vi "OE2012&OE2022_Query Multi Data.vi"(0 "VISA resource name":refnum<visa-resource-name>, 1 "OE2012&OE2022_\nQuery Multi Data":T2={"Query Type 1"=0, "Query Type 5"=32, "Query Type 4"=3, "Query Type 3"=2, "Query Type 2"=1, "Query Type 6"=36} {"Query Type 6" items=["X-Demod1", "Y-Demod1", "R-Demod1", "Theta-Demod1", "X-Demod2", "Y-Demod2", "R-Demod2", "Theta-Demod2", "X-Demod3", "Y-Demod3", "R-Demod3", "Theta-Demod3", "X-Demod4", "Y-Demod4", "R-Demod4", "Theta-Demod4", "X-Demod5", "Y-Demod5", "R-Demod5", "Theta-Demod5", "X-Demod6", "Y-Demod6", "R-Demod6", "Theta-Demod6", "X-Demod7", "Y-Demod7", "R-Demod7", "Theta-Demod7", "X-Demod8", "Y-Demod8", "R-Demod8", "Theta-Demod8", "Xnoisd-Demod1", "Ynoisd-Demod1", "Xnoisd-Demod5", "Ynoisd-Demod5", "Frequency-OSC1", "Frequency-OSC2", "AUXIN1", "AUXIN2", "AUXIN3", "AUXIN4", "Timestamps"]; "Query Type 2" items=["X-Demod1", "Y-Demod1", "R-Demod1", "Theta-Demod1", "X-Demod2", "Y-Demod2", "R-Demod2", "Theta-Demod2", "X-Demod3", "Y-Demod3", "R-Demod3", "Theta-Demod3", "X-Demod4", "Y-Demod4", "R-Demod4", "Theta-Demod4", "X-Demod5", "Y-Demod5", "R-Demod5", "Theta-Demod5", "X-Demod6", "Y-Demod6", "R-Demod6", "Theta-Demod6", "X-Demod7", "Y-Demod7", "R-Demod7", "Theta-Demod7", "X-Demod8", "Y-Demod8", "R-Demod8", "Theta-Demod8", "Xnoisd-Demod1", "Ynoisd-Demod1", "Xnoisd-Demod5", "Ynoisd-Demod5", "Frequency-OSC1", "Frequency-OSC2", "AUXIN1", "AUXIN2", "AUXIN3", "AUXIN4", "Timestamps"]; "Query Type 3" items=["X-Demod1", "Y-Demod1", "R-Demod1", "Theta-Demod1", "X-Demod2", "Y-Demod2", "R-Demod2", "Theta-Demod2", "X-Demod3", "Y-Demod3", "R-Demod3", "Theta-Demod3", "X-Demod4", "Y-Demod4", "R-Demod4", "Theta-Demod4", "X-Demod5", "Y-Demod5", "R-Demod5", "Theta-Demod5", "X-Demod6", "Y-Demod6", "R-Demod6", "Theta-Demod6", "X-Demod7", "Y-Demod7", "R-Demod7", "Theta-Demod7", "X-Demod8", "Y-Demod8", "R-Demod8", "Theta-Demod8", "Xnoisd-Demod1", "Ynoisd-Demod1", "Xnoisd-Demod5", "Ynoisd-Demod5", "Frequency-OSC1", "Frequency-OSC2", "AUXIN1", "AUXIN2", "AUXIN3", "AUXIN4", "Timestamps"]; "Query Type 4" items=["X-Demod1", "Y-Demod1", "R-Demod1", "Theta-Demod1", "X-Demod2", "Y-Demod2", "R-Demod2", "Theta-Demod2", "X-Demod3", "Y-Demod3", "R-Demod3", "Theta-Demod3", "X-Demod4", "Y-Demod4", "R-Demod4", "Theta-Demod4", "X-Demod5", "Y-Demod5", "R-Demod5", "Theta-Demod5", "X-Demod6", "Y-Demod6", "R-Demod6", "Theta-Demod6", "X-Demod7", "Y-Demod7", "R-Demod7", "Theta-Demod7", "X-Demod8", "Y-Demod8", "R-Demod8", "Theta-Demod8", "Xnoisd-Demod1", "Ynoisd-Demod1", "Xnoisd-Demod5", "Ynoisd-Demod5", "Frequency-OSC1", "Frequency-OSC2", "AUXIN1", "AUXIN2", "AUXIN3", "AUXIN4", "Timestamps"]; "Query Type 5" items=["X-Demod1", "Y-Demod1", "R-Demod1", "Theta-Demod1", "X-Demod2", "Y-Demod2", "R-Demod2", "Theta-Demod2", "X-Demod3", "Y-Demod3", "R-Demod3", "Theta-Demod3", "X-Demod4", "Y-Demod4", "R-Demod4", "Theta-Demod4", "X-Demod5", "Y-Demod5", "R-Demod5", "Theta-Demod5", "X-Demod6", "Y-Demod6", "R-Demod6", "Theta-Demod6", "X-Demod7", "Y-Demod7", "R-Demod7", "Theta-Demod7", "X-Demod8", "Y-Demod8", "R-Demod8", "Theta-Demod8", "Xnoisd-Demod1", "Ynoisd-Demod1", "Xnoisd-Demod5", "Ynoisd-Demod5", "Frequency-OSC1", "Frequency-OSC2", "AUXIN1", "AUXIN2", "AUXIN3", "AUXIN4", "Timestamps"]; "Query Type 1" items=["X-Demod1", "Y-Demod1", "R-Demod1", "Theta-Demod1", "X-Demod2", "Y-Demod2", "R-Demod2", "Theta-Demod2", "X-Demod3", "Y-Demod3", "R-Demod3", "Theta-Demod3", "X-Demod4", "Y-Demod4", "R-Demod4", "Theta-Demod4", "X-Demod5", "Y-Demod5", "R-Demod5", "Theta-Demod5", "X-Demod6", "Y-Demod6", "R-Demod6", "Theta-Demod6", "X-Demod7", "Y-Demod7", "R-Demod7", "Theta-Demod7", "X-Demod8", "Y-Demod8", "R-Demod8", "Theta-Demod8", "Xnoisd-Demod1", "Ynoisd-Demod1", "Xnoisd-Demod5", "Ynoisd-Demod5", "Frequency-OSC1", "Frequency-OSC2", "AUXIN1", "AUXIN2", "AUXIN3", "AUXIN4", "Timestamps"]}, 5 "Connection ID in":refnum<k5>, 7 "Remote Mode":u16(ring) items=["USB", "RS232", "GPIB", "Ethernet"], 11 "Error in (no error)":errorcluster caption="error out（no error）") -> (4 "VISA resource  out":refnum<visa-resource-name>, 6 "Connection ID out":refnum<k5>, 8 "Parameter Values":T1, 10 "Output String":string, 15 "Error out":errorcluster caption="error out")   [LabVIEW 2011]
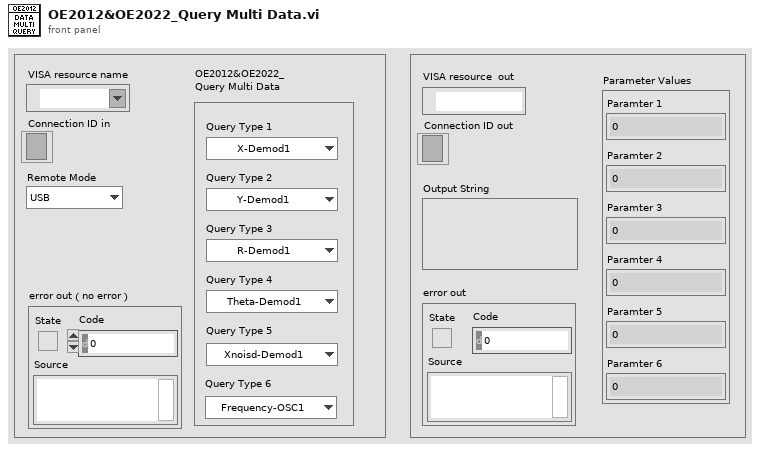
[diagram p1: front panel]
types:
  T1 = cluster{"Paramter 1":dbl, "Paramter 2":dbl, "Paramter 3":dbl, "Paramter 4":dbl, "Paramter 5":dbl, "Paramter 6":dbl}
  T2 = cluster{"Query Type 1":u16, "Query Type 5":u16, "Query Type 4":u16, "Query Type 3":u16, "Query Type 2":u16, "Query Type 6":u16}
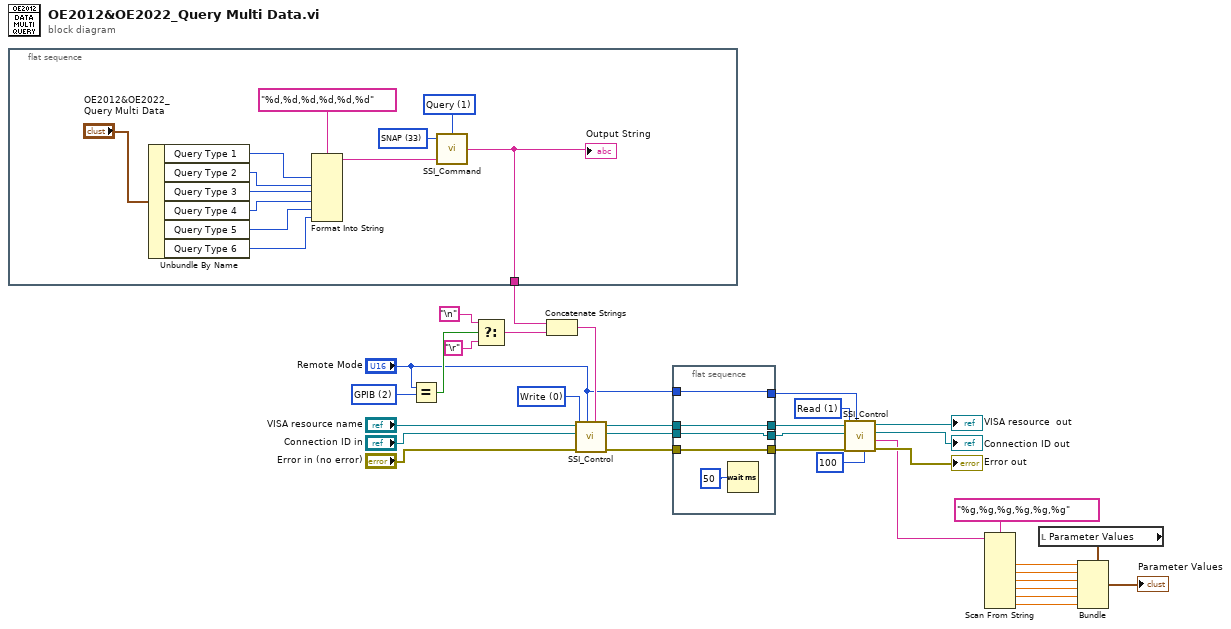
[diagram p0: block diagram]
diagram:
  w24 = u16 2 items=["USB", "RS232", "GPIB", "Ethernet"] ("Remote Mode")
  w29 = u16 1 items=["Write", "Read"] ("Control")
  w34 = u16 0 items=["Write", "Read"] ("Control")
  n1 = flat-sequence {
    tunnel: [w35] -> w13
    frame #0 {
      w46 = u16 33 items=["ISRC", "IGND", "ICPL", "ILIN", "PHAS", "FMOD", "RSLP", "FREQ", "SWPT", "SLLM", "SULM", "SSLL", "SSLG", "STLM", "SWRM", "IRNG", "SENS", "RMOD", "OFLT", "OFSL", "SYNC", "DMOD", "HARM", "DARB", "SWVT", "SLVL", "SVLL", "SVUL", "SVSL", "SVSG", "SVTM", "SVRM", "RALL", "SNAP", "OUTP", "OAUX", "COUT", "CAUX", "COFP", "CEXP", "FPOP", "OEXP", "*IDN", "*RST", "OVLD", "INOV", "GNOV", "*PLL", "SSET", "RSET", "AGAN", "APHS", "ARSV", "ASCL", "EQCD", "EQCS", "SPED", "SRAT", "SLEN", "SSLE", "STRG", "SPRM", "STRD", "PAUS", "RSET", "SPTS", "TRCA", "TEMP", "RSTU", "INHZ", "DEQU", "SADD", "ARNG", "CSPE", "ISRCD", "IGNDD", "ICPLD", "ILIND", "PHASD", "FMODD", "RSLPD", "FREQD", "SWPTD", "SLLMD", "SULMD", "SSLLD", "SSLGD", "STLMD", "SWRMD", "SENSD", "RMODD", "OFLTD", "OFSLD", "SYNCD", "HARMD", "EQCDD", "EQCSD", "SNAPD", "OUTPD", "SWVTD", "SLVLD", "SVLLD", "SVULD", "SVSLD", "SVSGD", "SVTMD", "SVRMD", "SVDCD", "ARSVD", "AGAND", "APHSD", "ASCLD", "FPOPD", "CAUXD", "OEXPD", "SPEDD", "SRATD", "SLEND", "SSLED", "STRGD", "SPRMD", "STRDD", "PAUSD", "RESTD", "SPTSD", "TRCAD", "*IDND", "*RSTD", "INOVD", "GNOVD", "*PLLD", "SSETD", "RSETD", "RALLD"] ("Command Type")
      w45 = u16 1 items=["Set", "Query"] ("Opera")
      n2 = Unbundle By Name("OE2012&OE2022_\nQuery Multi Data") -> ("Query Type 1"=w43:u16, "Query Type 2"=w42:u16, "Query Type 3"=w41:u16, "Query Type 4"=w40:u16, "Query Type 5"=w39:u16, "Query Type 6"=w38:u16)
      n3 = Format Into String(format string="%d,%d,%d,%d,%d,%d" ("格式字符串"), w43, w42, w41, w40, w39, w38) -> (resulting string=w36:string)  [unwired: 2 in, 1 out]
      n4 = call "SSI_Command.vi"("Opera"=w45, "Paramter"=w36, "Command Type"=w46) -> ("Output string"=w35:string)  [unwired: 1 in]
      "Output String" <- w35
    }
  }
  n5 = Equal?(x="Remote Mode", y=w24) -> (x = y?=w19:bool)
  n6 = Select(t="\n", s=w19, f="\r") -> (s? t:f=w22:string)
  n7 = Concatenate Strings(w13, w22) -> (w20:string)
  n8 = call "SSI_Control.vi"("Write Buffer"=w20, "Remote Mode"="Remote Mode", "Error in (no error)"="Error in (no error)", "Control"=w34, "Connection ID in"="Connection ID in", "VISA resource name"="VISA resource name") -> ("Error out"=w32:errorcluster, "Connection ID out"=w3:refnum<k5>, "VISA resource  out"=w33:refnum<visa-resource-name>)  [unwired: 2 in, 1 out]
  n9 = flat-sequence {
    tunnel: w33 -> [w51]
    tunnel: w32 -> [w50]
    tunnel: [w51] -> w31
    tunnel: [w50] -> w30
    tunnel: [w48] -> w28
    tunnel: "Remote Mode" -> [w48]
    tunnel: w3 -> [w47]
    tunnel: [w47] -> w2
    frame #0 {
      n10 = Wait (ms)(milliseconds to wait=u32 50 ("等待时间（毫秒）")) -> ()  [unwired: 1 out]
    }
  }
  n11 = call "SSI_Control.vi"("Tineout"=100, "Remote Mode"=w28, "Error in (no error)"=w30, "Control"=w29, "Connection ID in"=w2, "VISA resource name"=w31) -> ("Error out"=→"Error out":errorcluster, "Read Buffer"=w16:string, "Connection ID out"=→"Connection ID out":refnum<k5>, "VISA resource  out"=→"VISA resource  out":refnum<visa-resource-name>)  [unwired: 2 in]
  n12 = Scan From String(format string="%g,%g,%g,%g,%g,%g" ("格式字符串"), input string=w16) -> (output 1=w12:dbl, output 2=w11:dbl, output 3=w10:dbl, output 4=w9:dbl, output 5=w8:dbl, output 6=w5:dbl)  [unwired: 8 in, 3 out]
  n13 = local read "Parameter Values"() -> (w6:T1)
  n14 = Bundle(cluster=w6, "Paramter 1"=w12, "Paramter 2"=w11, "Paramter 3"=w10, "Paramter 4"=w9, "Paramter 5"=w8, "Paramter 6"=w5) -> (→"Parameter Values":T1)
